vi "Utility_Detect Button Change.vi"(11 "HW_Joystick_Buttons":bool[](array[boolean])) -> (0 "Toggle On Rising Out":bool[](array[boolean]), 1 "Falling Out":bool[](array[boolean]), 2 "Rising Out":bool[](array[boolean]), 3 "Value Out":bool[](array[boolean]), 4 "Toggle On Falling Out":bool[](array[boolean]))   [LabVIEW 2020]
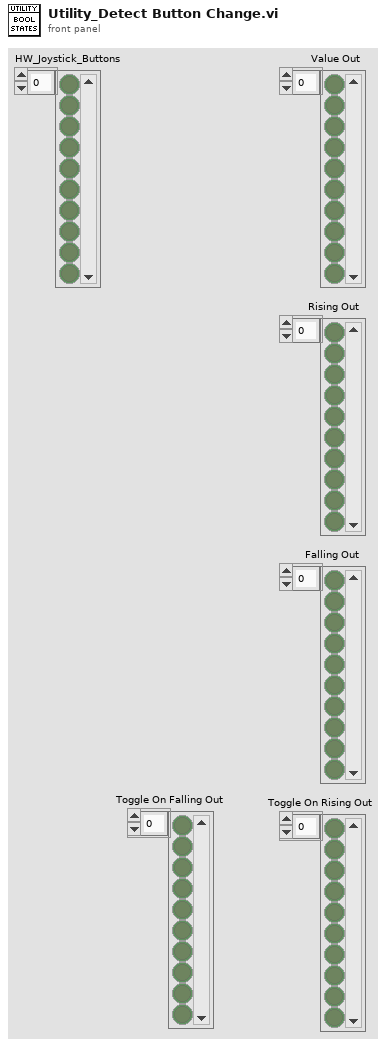
[diagram p1: front panel]
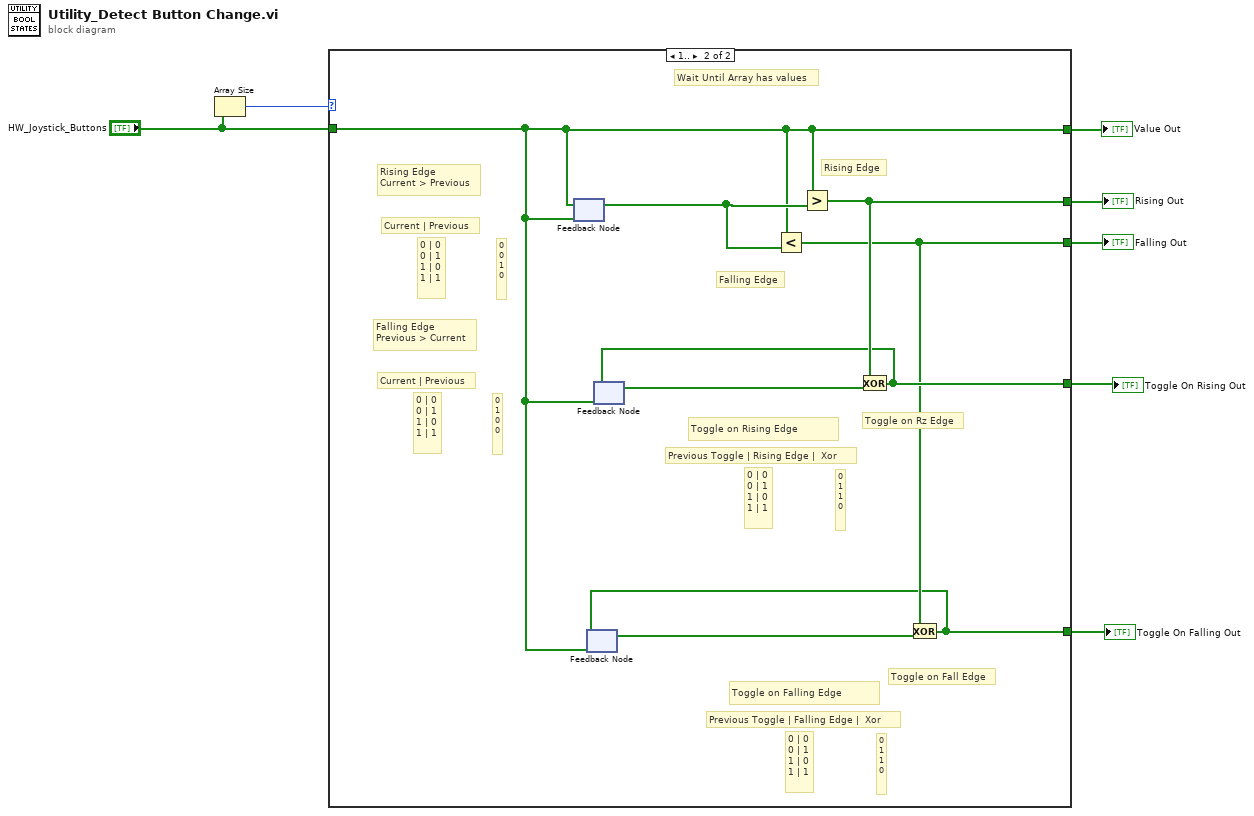
[diagram p0: block diagram]
diagram:
  n1 = Array Size(array="HW_Joystick_Buttons") -> (size(s)=w2:i32)
  n2 = case shown="1.." w2 {
    tunnel: [_ w15] -> w7
    tunnel: [_ w14] -> w6
    tunnel: [_ w12] -> w5
    tunnel: [_ w11] -> w4
    tunnel: "HW_Joystick_Buttons" -> [w8 w9]
    tunnel: [w8 w9] -> w1
    frame ..0 {
      # "No array values"
    }
    frame 1.. {
      # "Toggle on Falling Edge"
      # "0\n1\n1\n0"
      # "0 | 0 \n0 | 1\n1 | 0\n1 | 1"
      # "Previous Toggle | Falling Edge |  Xor"
      # "0\n1\n0\n0"
      # "0 | 0 \n0 | 1\n1 | 0\n1 | 1"
      # "Current | Previous"
      # "Falling Edge \nPrevious > Current"
      # "Toggle on Fall Edge"
      # "0\n0\n1\n0"
      # "0 | 0 \n0 | 1\n1 | 0\n1 | 1"
      # "Current | Previous"
      # "Rising Edge \nCurrent > Previous"
      # "Toggle on Rz Edge"
      # "Toggle on Rising Edge"
      # "0\n1\n1\n0"
      # "0 | 0 \n0 | 1\n1 | 0\n1 | 1"
      # "Previous Toggle | Rising Edge |  Xor"
      # "Falling Edge"
      # "Rising Edge"
      # "Wait Until Array has values"
      n3 = feedback #1(w9) -> (w10:bool[])
      n4 = feedback-in #1(w9) -> ()
      n5 = feedback #2(w9) -> (w13:bool[])
      n6 = feedback #3(w9) -> (w16:bool[])
      n7 = Less?(x=w9, y=w10) -> (x < y?=w12:bool[])
      n8 = Greater?(x=w9, y=w10) -> (0:w15:bool[])
      n9 = Exclusive Or(1:w16, 2:w15) -> (0:w14:bool[])
      n10 = feedback-in #3(w14) -> ()
      n11 = Exclusive Or(1:w13, 2:w12) -> (0:w11:bool[])
      n12 = feedback-in #2(w11) -> ()
    }
  }
  "Rising Out" <- w7
  "Value Out" <- w1
  "Falling Out" <- w5
  "Toggle On Rising Out" <- w6
  "Toggle On Falling Out" <- w4
